vi "Transformation(R+d).vi"(2 "Translation":dbl[](array[numeric]), 3 "rotation matrix":T1) -> (1 "Transformation matrix":T1)   [LabVIEW 2024]
uses:
  <vilib>/Analysis/Matrix/Datatypes/RealMatrix.ctl
  <vilib>/Analysis/Matrix/NI_Matrix.lvlib
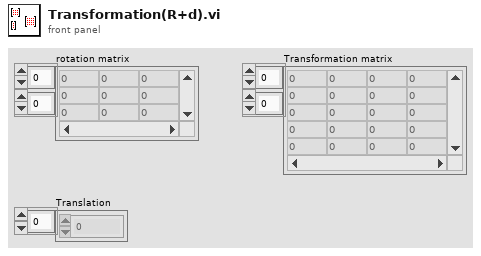
[diagram p1: front panel]
types:
  T1 = typedef "NI_Matrix.lvlib/RealMatrix.ctl" = dbl[][]
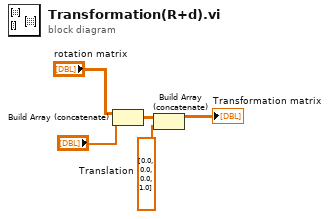
[diagram p0: block diagram]
diagram:
  n1 = Build Array (concatenate)("rotation matrix", "Translation") -> (w4:T1)
  n2 = Build Array (concatenate)(w4, dbl[] [0.0, 0.0, 0.0, 1.0] ("element")) -> (→"Transformation matrix":T1)
